vi "UTIL Extract Sleep Features.vi"(8 "Error In":errorcluster, 10 "Components In":T1) -> (0 "Error Out":errorcluster, 1 "Hi:Lo":dbl, 2 "Delta:Theta":dbl, 3 "Components Out":T1)   [LabVIEW 2017]
doc: "Given a set of EEG Components, this returns two ratios to be used a sleep features: Delta-Theta Ratio and the High-Low Ratio.\n\nDelta-Theta Ratio: (Delta Low + Delta High)/Theta\nHigh-Low Ratio: (Alpha + Beta + Gamma)/(Delta + Theta)\n\nInputs:\n EEG Components In Cluster of Dbl, TYPE EEG Component\n Error In\nOutputs:\n EEG Components Out Passthrough\n Delta:Theta Dbl\n Hi:Lo Dbl\n Error Out"
uses:
  Types/TYPE EEG Components.ctl
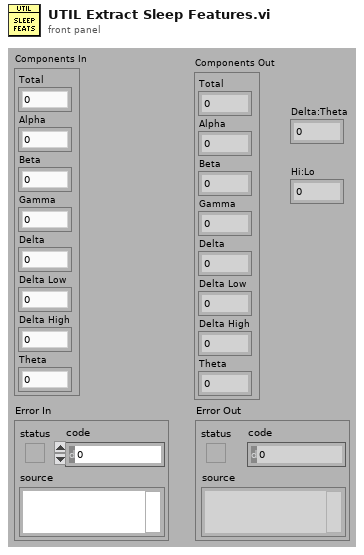
[diagram p1: front panel]
types:
  T1 = typedef "TYPE EEG Components.ctl" = cluster{"Total":dbl, "Alpha":dbl, "Beta":dbl, "Gamma":dbl, "Delta":dbl, "Delta Low":dbl, "Delta High":dbl, "Theta":dbl}
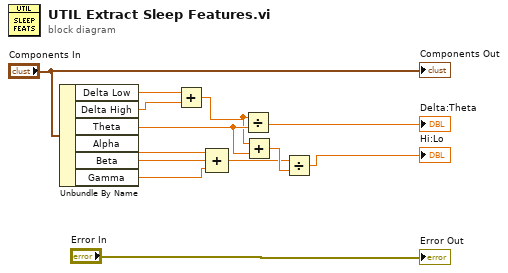
[diagram p0: block diagram]
diagram:
  n1 = Unbundle By Name("Components In") -> ("Delta Low"=w6:dbl, "Delta High"=w7:dbl, "Theta"=w10:dbl, "Alpha"=w2:dbl, "Beta"=w3:dbl, "Gamma"=w4:dbl)
  n2 = Add(x=w6, y=w7) -> (x+y=w5:dbl)
  n3 = Compound Arithmetic op=ADD(w2, w3, w4) -> (w1:dbl)
  n4 = Divide(x=w5, y=w10) -> (x/y=→"Delta:Theta":dbl)
  n5 = Add(x=w5, y=w10) -> (x+y=w9:dbl)
  n6 = Divide(x=w1, y=w9) -> (x/y=→"Hi:Lo":dbl)
  "Error Out" <- "Error In"
  "Components Out" <- "Components In"
